vi "checkSettingsClass.vi"(8 "error in (no error)":errorcluster, 11 "Tapedrive_ESP301 in":refnum<class "Tapedrive_ESP301.lvclass">) -> (0 "error in (no error) 2":errorcluster, 1 "forwardaxis":i16, 2 "settings needed":bool, 3 "spreadsheet string":string, 4 "Tension":T1)   [LabVIEW 2013, in "Tapedrive_ESP301.lvclass"]
uses:
  Tapedrive_ESP301.lvclass
  shared/OnOffTypeDef.ctl
  Tapedrive_ESP301.lvclass/Tapedrive_ESP301.ctl
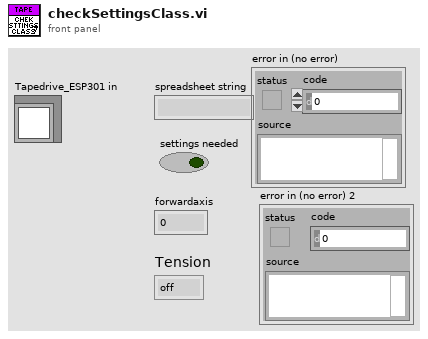
[diagram p1: front panel]
types:
  T1 = typedef "OnOffTypeDef.ctl" = enum16{"off", "on"}
  T2 = cluster{"Axis 1":cluster{"Value":dbl, "Min":dbl, "Max":dbl, "StepSize":dbl, "Tolerance":dbl, "ValueActual":dbl}, "Axis 2":cluster{"Value":dbl, "Min":dbl, "Max":dbl, "StepSize":dbl, "Tolerance":dbl, "ValueActual":dbl}}
  T3 = cluster{"Axis 1":cluster{"Value":dbl, "Min":dbl, "Max":dbl, "StepSize":dbl, "Tolerance":dbl, "ValueActual":dbl}, "Axis 2":cluster{"Value":dbl, "Min":dbl, "Max":dbl, "StepSize":dbl, "Tolerance":dbl, "ValueActual":dbl}}[]
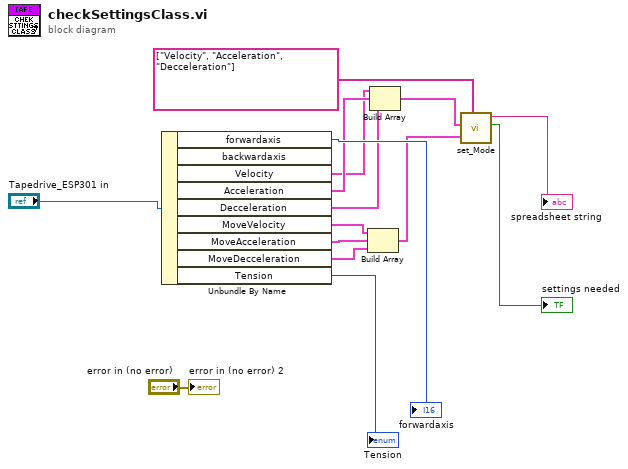
[diagram p0: block diagram]
diagram:
  n1 = Unbundle By Name("Tapedrive_ESP301 in") -> ("forwardaxis"=→"forwardaxis":i16, "Velocity"=w3:T2, "Acceleration"=w4:T2, "Decceleration"=w5:T2, "MoveVelocity"=w6:T2, "MoveAcceleration"=w7:T2, "MoveDecceleration"=w8:T2, "Tension"=→"Tension":T1)  [unwired: 1 out]
  n2 = Build Array(w6, w7, w8) -> (w10:T3)
  n3 = Build Array(w3, w4, w5) -> (w9:T3)
  n4 = call "set_Mode.vi"("Array"=w10, "Array 3"=string[] ["Velocity", "Acceleration", "Decceleration"], "Array 2"=w9) -> ("settings needed"=→"settings needed":bool, "spreadsheet string"=→"spreadsheet string":string)  [unwired: 7 in]
  "error in (no error) 2" <- "error in (no error)"
